vi "Initialize.vi"(8 "error in (no error)":errorcluster, 9 "PPLs Folder Path":path, 10 "INI File Path":path, 11 "Device":string) -> (0 "error out":errorcluster, 3 "LiDAR out":refnum<class "LiDAR.lvclass">)   [LabVIEW 2018, in "LiDAR.lvlib" / "LiDAR.lvclass"]
uses:
  LiDAR.lvclass
  LiDAR.lvclass/LiDAR.ctl
  PPLs/Configuration/Configuration.lvlibp/Configuration.lvclass
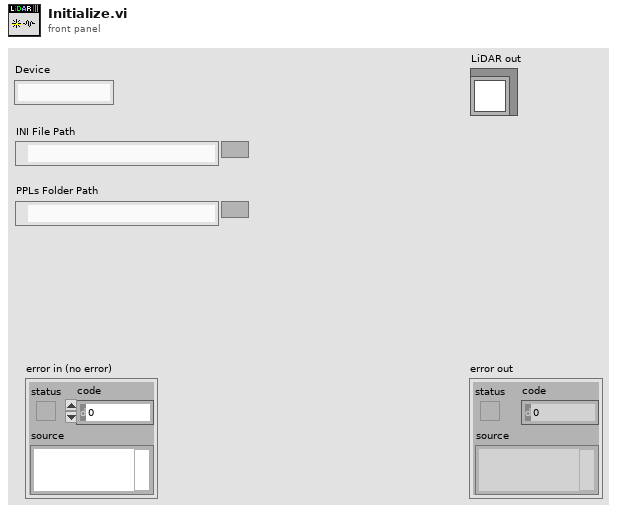
[diagram p1: front panel]
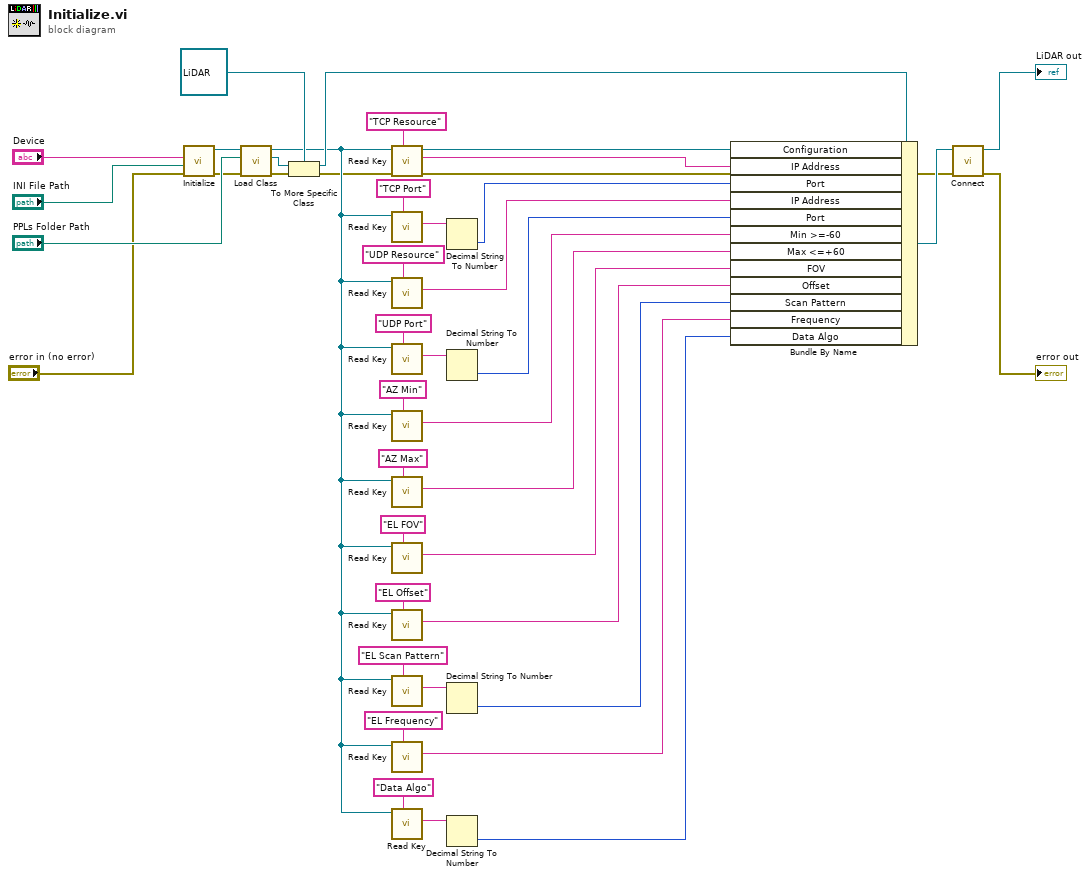
[diagram p0: block diagram]
diagram:
  n1 = call "Initialize.vi"("error in"="error in (no error)", "INI File Path"="INI File Path", "Device"="Device") -> ("error out"=w34:errorcluster, "Configuration out"=w32:refnum<class "Configuration.lvclass">)  [unwired: 7 in]
  n2 = call "Load Class.vi"("error in"=w34, "PPLs Folder Path"="PPLs Folder Path", "Configuration in"=w32) -> ("error out"=w42:errorcluster, "Class out"=w41:refnum<class>, "Configuration out"=w18:refnum<class "Configuration.lvclass">)  [unwired: 6 in]
  n3 = To More Specific Class(target class=refnum<class "LiDAR.lvclass"> refnum ("LiDAR in"), reference=w41, error in=w42) -> (specific class reference=w39:refnum<class "LiDAR.lvclass">, error out=w1:errorcluster)
  n4 = call "Read Key.vi"("Key:"="TCP Resource", "Configuration in"=w18) -> ("Value"=w13:string, "Configuration out"=w36:refnum<class "Configuration.lvclass">)  [unwired: 7 in, 1 out]
  n5 = call "Read Key.vi"("Key:"="TCP Port", "Configuration in"=w18) -> ("Value"=w16:string)  [unwired: 7 in, 2 out]
  n6 = call "Read Key.vi"("Key:"="UDP Resource", "Configuration in"=w18) -> ("Value"=w14:string)  [unwired: 7 in, 2 out]
  n7 = call "Read Key.vi"("Key:"="UDP Port", "Configuration in"=w18) -> ("Value"=w12:string)  [unwired: 7 in, 2 out]
  n8 = call "Read Key.vi"("Key:"="AZ Min", "Configuration in"=w18) -> ("Value"=w10:string)  [unwired: 7 in, 2 out]
  n9 = call "Read Key.vi"("Key:"="AZ Max", "Configuration in"=w18) -> ("Value"=w9:string)  [unwired: 7 in, 2 out]
  n10 = call "Read Key.vi"("Key:"="EL FOV", "Configuration in"=w18) -> ("Value"=w8:string)  [unwired: 7 in, 2 out]
  n11 = call "Read Key.vi"("Key:"="EL Offset", "Configuration in"=w18) -> ("Value"=w7:string)  [unwired: 7 in, 2 out]
  n12 = call "Read Key.vi"("Key:"="EL Scan Pattern", "Configuration in"=w18) -> ("Value"=w6:string)  [unwired: 7 in, 2 out]
  n13 = call "Read Key.vi"("Key:"="EL Frequency", "Configuration in"=w18) -> ("Value"=w4:string)  [unwired: 7 in, 2 out]
  n14 = call "Read Key.vi"("Key:"="Data Algo", "Configuration in"=w18) -> ("Value"=w3:string)  [unwired: 7 in, 2 out]
  n15 = Decimal String To Number(string=w16) -> (number=w15:i32)  [unwired: 2 in, 1 out]
  n16 = Decimal String To Number(string=w12) -> (number=w11:i32)  [unwired: 2 in, 1 out]
  n17 = Decimal String To Number(string=w6) -> (number=w5:i32)  [unwired: 2 in, 1 out]
  n18 = Decimal String To Number(string=w3) -> (number=w2:i32)  [unwired: 2 in, 1 out]
  n19 = Bundle By Name(cluster=w39, "Configuration"=w36, "IP Address"=w13, "Port"=w15, "IP Address"=w14, "Port"=w11, "Min >=-60"=w10, "Max <=+60"=w9, "FOV"=w8, "Offset"=w7, "Scan Pattern"=w5, "Frequency"=w4, "Data Algo"=w2) -> (w17:refnum<class "LiDAR.lvclass">)
  n20 = call-dynamic "Connect.vi"("error in (no error)"=w1, "LiDAR in"=w17) -> ("error out"=→"error out":errorcluster, "LiDAR out"=→"LiDAR out":refnum<class "LiDAR.lvclass">)  [unwired: 8 in]
